vi "GetParam.vi"(8 "error in (no error)":errorcluster caption="entrée d'erreur (pas d'erreur)", 11 "20newsgroups.lvclass":refnum<class "20newsgroups.lvclass">) -> (0 "error out":errorcluster caption="sortie d'erreur", 2 "fetch_20newsgroups":T1={"subset"="train", "categories"=["None"], "shuffle"=TRUE, "random_state"=42, "remove"=[], "download_if_missing"=TRUE, "Returns"="Data"} {"random_state" min=-1}, 3 "20newsgroups.lvclass":refnum<class "20newsgroups.lvclass">)   [LabVIEW 2020, in "20newsgroups.lvclass"]
doc: "Get parameters"
uses:
  20newsgroups.lvclass
  20newsgroups.lvclass/20newsgroups.ctl
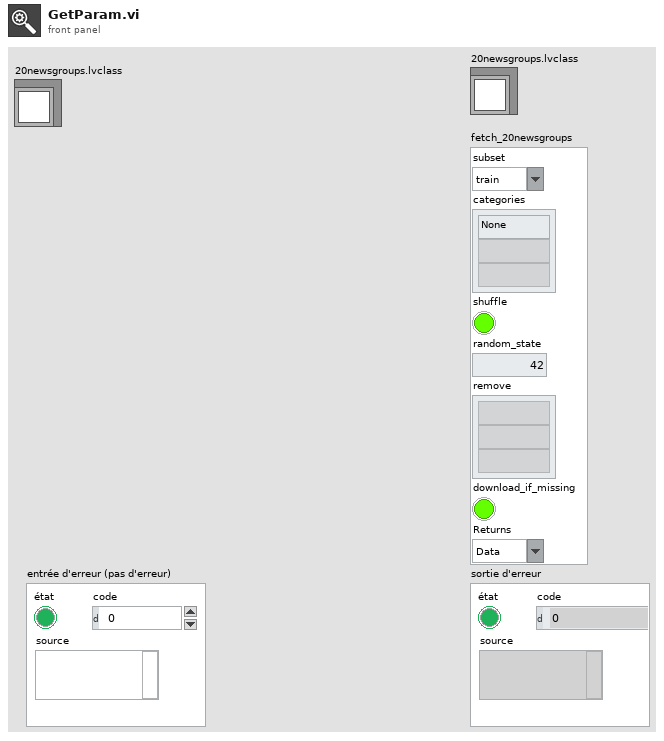
[diagram p1: front panel]
types:
  T1 = cluster{"subset":string, "categories":string[], "shuffle":bool, "random_state":i32, "remove":string[], "download_if_missing":bool, "Returns":string}
  T2 = cluster{"subset":string, "categories":string[], "shuffle":bool, "random_state":i32, "remove":string[], " download_if_missing ":bool, "Returns":string}
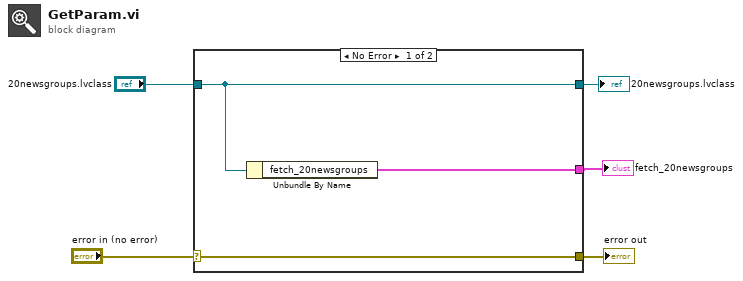
[diagram p0: block diagram]
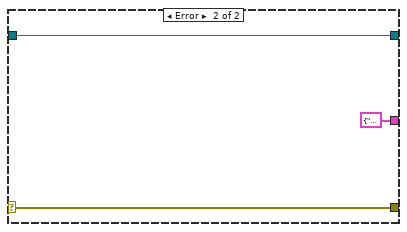
[diagram p2: hidden frame]
diagram:
  n1 = case shown="No Error" "error in (no error)" {
    selector: "error in (no error)" -> [w8 w10]
    tunnel: [w8 w10] -> w4
    tunnel: [w7 w11] -> w1
    tunnel: "20newsgroups.lvclass" -> [w7 w11]
    tunnel: [w6 T2 {"subset"="", "categories"=[], "shuffle"=FALSE, "random_state"=0, "remove"=[], " download_if_missing "=FALSE, "Returns"=""} ("fetch_20newsgroups")] -> w3
    frame No Error {
      n2 = Unbundle By Name(w7) -> ("fetch_20newsgroups"=w6:T2)
    }
    frame Error {
    }
  }
  "error out" <- w4
  "fetch_20newsgroups" <- w3
  "20newsgroups.lvclass" <- w1
